vi "SDM Check Global Channel Ports.vi"(0 "Global Channel In":refnum<k21>, 11 "error in (no error)":errorcluster) -> (4 "Global Channel Out":refnum<k21>, 15 "error out":errorcluster)   [LabVIEW 2021, in "DAQ_Static Digital State Measurement.lvlib"]
doc: "Checks for the presence of port in the global channel input and throws the required error when identified."
uses:
  DAQ_Static Digital State Measurement.lvlib
  <vilib>/Utility/error.llb/Error Cluster From Error Code.vi
  <vilib>/ErrorRing/Error Ring.xnode
  <resource>/objmgr/daqmx.rc
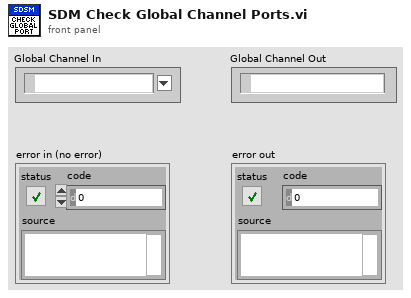
[diagram p1: front panel]
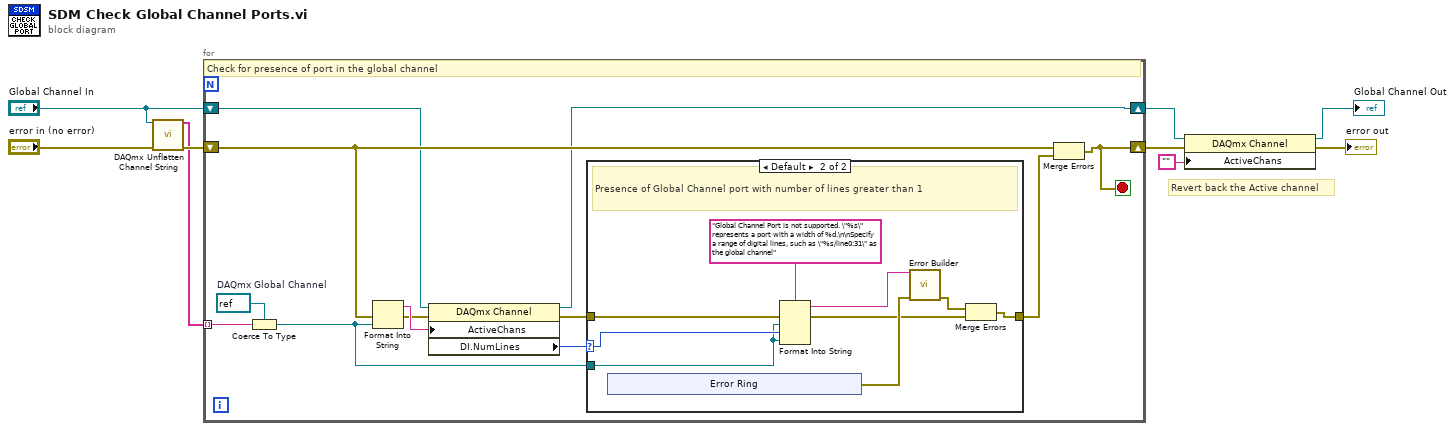
[diagram p0: block diagram]
diagram:
  # "Revert back the Active channel"
  n1 = call <vilib>:"DAQmx Unflatten Channel String.vi"("names in"="Global Channel In", "error in"="error in (no error)") -> ("names out"=w7:string[], "error out"=w8:errorcluster)  [unwired: 12 in]
  n2 = for {
    tunnel: w7 -> [w21] mode=indexing
    shift-right: [w18] -> w4
    shift-left: w8 -> [w14]
    shift-right: [w10] -> w6
    shift-left: "Global Channel In" -> [w11]
    stop <- w18 stop-if-true
    w20 = refnum<k21> refnum  # DAQmx Global Channel
    # "Check for presence of port in the global channel"
    n3 = Coerce To Type(0:w21, 1:w20) -> (2:w15:refnum<k21>)
    n4 = Format Into String(error in=w14, w15) -> (resulting string=w13:string, error out=w12:errorcluster)  [unwired: 2 in]
    n5 = property class="DAQmx Channel"(reference=w11, error in=w12, "ActiveChans"=w13) -> (reference out=w10:refnum<k21>, error out=w16:errorcluster, "DI.NumLines"=w17:u32)
    n6 = case shown="Default" w17 {
      selector: w17 -> [_ w25]
      tunnel: [w22 w26] -> w19
      tunnel: w15 -> [_ w24]
      tunnel: w16 -> [w22 w27]
      frame 1 {
        # "The current active channel is a singe digital line"
      }
      frame Default {
        # "Presence of Global Channel port with number of lines greater than 1"
        n7 = xnode "Error Ring"() -> ("error out"=w30:errorcluster)
        n8 = Format Into String(format string="Global Channel Port is not supported. \"%s\" represents a port with a width of %d.\n\nSpecify a range of digital lines, such as \"%s/line0:31\" as the global channel" ("error message (\"\")"), error in=w27, w24, w25, w24) -> (resulting string=w31:string, error out=w28:errorcluster)  [unwired: 1 in]
        n9 = call "Error Builder.vi"("Error String"=w31, "Error In"=w30) -> ("Error Out"=w29:errorcluster)  [unwired: 13 in]
        n10 = Merge Errors(w29, w28) -> (w26:errorcluster)
      }
    }
    n11 = Merge Errors(w14, w19) -> (w18:errorcluster)
  }
  n12 = property class="DAQmx Channel"(reference=w6, error in=w4, "ActiveChans"="") -> (reference out=→"Global Channel Out":refnum<k21>, error out=→"error out":errorcluster)
